vi "Get TSM Site Context Index.vi"(0 "Semiconductor Module Context":T1, 5 "Site Number":i32, 11 "error in (no error)":errorcluster) -> (4 "index of Site TSM Context":i32, 15 "error out":errorcluster)   [LabVIEW 2023, in "RFCalAndFixtureCharact.Common.lvlib" / "Path Group.lvclass"]
uses:
  Path Group.lvclass
  <vilib>/NI_TestStand_SemiconductorModule/NI_TestStand_Semiconductor_Module.lvlibp/PinMap/General/SemiconductorModuleContext.ctl
  7af278ce-5371-4c9a-a082-b83abced347c.vi
  <vilib>/Comparison/Equal/Equal Functor/Equal Functor.lvclass
  <vilib>/NI_TestStand_SemiconductorModule/NI_TestStand_Semiconductor_Module.lvlibp
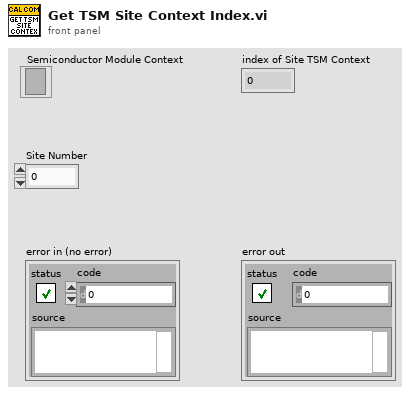
[diagram p1: front panel]
types:
  T1 = typedef "NI_TestStand_Semiconductor_Module.lvlibp/SemiconductorModuleContext.ctl" = refnum<k7>
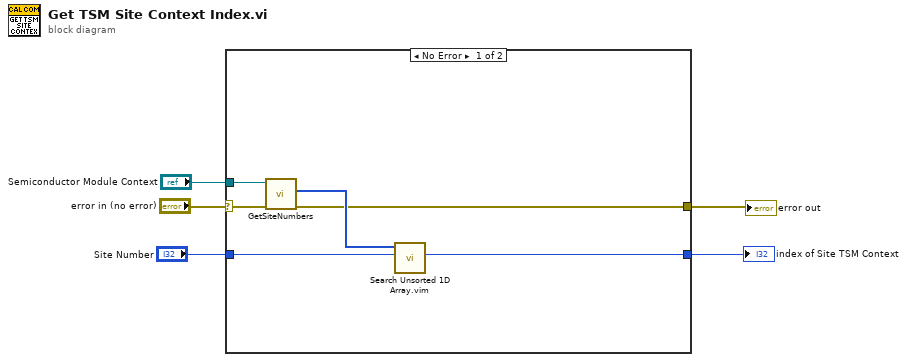
[diagram p0: block diagram]
diagram:
  n1 = case shown="No Error" "error in (no error)" {
    selector: "error in (no error)" -> [w10 w12]
    tunnel: "Semiconductor Module Context" -> [w11 _]
    tunnel: "Site Number" -> [w8 _]
    tunnel: [w7 w12] -> w2
    tunnel: [w6 _] -> w1
    frame No Error {
      n2 = call <vilib>:"GetSiteNumbers.vi"("error in (no error)"=w10, "Semiconductor Module Context"=w11) -> ("error out"=w7:errorcluster, "Site Numbers"=w9:i32[])  [unwired: 6 in, 2 out]
      n3 = call "Search Unsorted 1D Array.vim"("element"=w8, "unsorted 1D array"=w9) -> ("index of element"=w6:i32)  [unwired: 9 in]
    }
    frame Error {
    }
  }
  "error out" <- w2
  "index of Site TSM Context" <- w1
